vi "ziSweeperUtilEX.vi"(0 "Handle In":T1 {"Handle" format="0x%08x"; "Conn" format="0x%08x"}, 1 "Input Demods (0)":u16[](array[numeric])=[0], 2 "Oscillator (0)":u16, 3 "Order (4)":i32=4, 4 "Harmonic (1=fundamental)":i32=1 min=1 max=66000, 5 "Error In":errorcluster, 6 "Start (Hz)":dbl=10.0 format="%#_12p", 7 "average":u16, 8 "Stop (Hz)":dbl=10000.0 format="%#_12p", 9 "Precision (Low)":i32(ring)=5 items=["Low"=5, "Medium"=15, "High"=50], 10 "Steps (#)":i32=2, 11 "Min 1-w Damping (40dB)":dbl=40.0, 12 "Log Sweep (true)":bool=TRUE, 13 "Bandwith (-1=auto)":dbl=-1.0 format="%#_12p") -> (14 "Handle Out":T1 {"Handle" format="0x%08x"; "Conn" format="0x%08x"}, 15 "Output (F,X1,Y1,X2,Y2,...,Vo)":dbl[][](array[numeric]) format="%#_4p", 19 "Error Out":errorcluster)   [LabVIEW 2009, in "Zurich Instruments LabOne.lvlib"]
doc: "This utility configures an sweeper instance and returns after a complete single run the data recordered."
uses:
  <instrlib>/Zurich Instruments LabOne/Zurich Instruments LabOne.lvlib
  <instrlib>/Zurich Instruments LabOne/Public/ziTypeHandle.ctl
  <instrlib>/Zurich Instruments LabOne/Public/Modules/ziTypeModEnum.ctl
  <instrlib>/Zurich Instruments LabOne/Public/Modules/ziModSetValueDoubleArray.vi
  <instrlib>/Zurich Instruments LabOne/Public/Modules/ziModSetValueBinaryArray.vi
  <instrlib>/Zurich Instruments LabOne/Public/Configure/ziSetValueDouble.vi
  <instrlib>/Zurich Instruments LabOne/Public/Modules/ziModGetSweeperData.vi
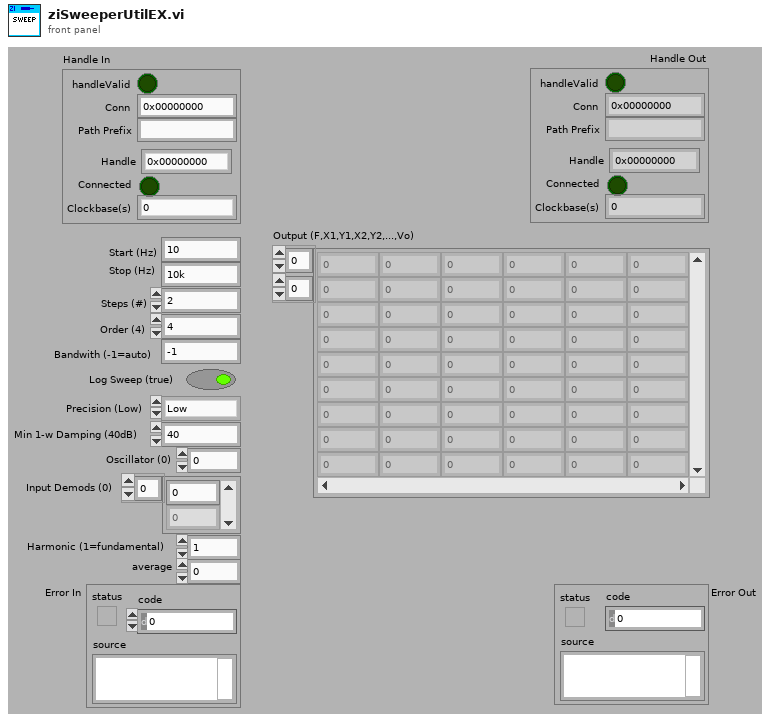
[diagram p1: front panel]
types:
  T1 = typedef "Zurich Instruments LabOne.lvlib/ziTypeHandle.ctl" = cluster{"handleValid":bool, "Conn":u64, "Path Prefix":string, "Handle":u64, "Connected":bool, "Clockbase(s)":dbl}
  T2 = typedef "Zurich Instruments LabOne.lvlib/ziTypeModEnum.ctl" = u16
  T3 = typedef "Zurich Instruments LabOne.lvlib/ziTypeModHandle.ctl" = cluster{"handleValid":bool, "Conn":u64, "ModHandle":u64, "moduleID":string, "Path Prefix":string}
  T4 = typedef "Zurich Instruments LabOne.lvlib/ziTypeModResults.ctl" = cluster{"PathArray":string[], "ValueType":T5, "NoOfResults":u64, "ziGenericHeader":T6[]}
  T5 = typedef "Zurich Instruments LabOne.lvlib/ziTypePollType.ctl" = enum16{"NONE", "DOUBLE_DATA", "INTEGER_DATA", "DEMOD_SAMPLE", "SCOPE_WAVE_HF2", "AUXIN_SAMPLE", "DIO_SAMPLE", "BYTE_ARRAY", "PWA_WAVE", "9", "10", "11", "12", "13", "14", "15", "TREE_CHANGE_DEPRI", "17", "ERROR", "19", "20", "21", "22", "23", "24", "25", "26", "27", "28", "29", "30", "31", "DOUBLE_DATA_TS", "INTEGER_DATA_TS", "34", "SCOPE_WAVE", "SCOPE_WAVE_EX", "37", "BYTE_ARRAY_TS", "39", "40", "41", "42", "43", "44", "45", "CNT_DATA", "47", "TREE_CHANGE", "49", "50", "51", "52", "53", "54", "55", "56", "57", "58", "59", "60", "61", "62", "63", "SWEEPER_DATA", "SPECTRUM_DATA", "ADVISOR_DATA", "VECTOR_DATA", "IMP_DATA"}
  T6 = typedef "Zurich Instruments LabOne.lvlib/ziTypeModGenericHeader.ctl" = cluster{"HeaderType":enum8{"HEADER_TYPE_NONE", "HEADER_TYPE_SWTRIGGER", "HEADER_TYPE_SWEEPER"}, "SampleFormat":u8, "SystemTime":timestamp, "CreatedTimeStamp":u64, "ChangedTimeStamp":u64, "Flags":u32, "ChunkSizeBytes":u64, "Name":string, "Status":u32, "GroupIndex":u32, "Color":u32, "ActiveRow":u32, "TriggerNumber":u64, "GridRows":u32, "GridCols":u32, "GridMode":u32, "GridOperation":u32, "GridDirection":u32, "GridRepetitions":u32, "GridColDelta":dbl, "GridColOffset":dbl, "GridRowDelta":dbl, "GridRowOffset":dbl, "Bandwidth":dbl, "Center":dbl, "Nenbw":dbl}
  T7 = typedef "Zurich Instruments LabOne.lvlib/ziTypeModSweeperDemodWave.ctl" = cluster{"timestamp":u64, "sampleCount":u64, "flags":u8, "sampleFormat":u8, "sweepMode":u8, "bandwidthMode":u8, "count":u64[], "settimestamp":u64[], "nexttimestamp":u64[], "grid":dbl[], "bandwidth":dbl[], "tc":dbl[], "tcmeas":dbl[], "settling":dbl[], "x":dbl[], "xstddev":dbl[], "xpwr":dbl[], "y":dbl[], "ystddev":dbl[], "ypwr":dbl[], "r":dbl[], "rstddev":dbl[], "rpwr":dbl[], "phase":dbl[], "phasestddev":dbl[], "phasepwr":dbl[], "frequency":dbl[], "frequencystddev":dbl[], "frequencypwr":dbl[], "auxin0":dbl[], "auxin0stddev":dbl[], "auxin0pwr":dbl[], "auxin1":dbl[], "auxin1stddev":dbl[], "auxin1pwr":dbl[]}
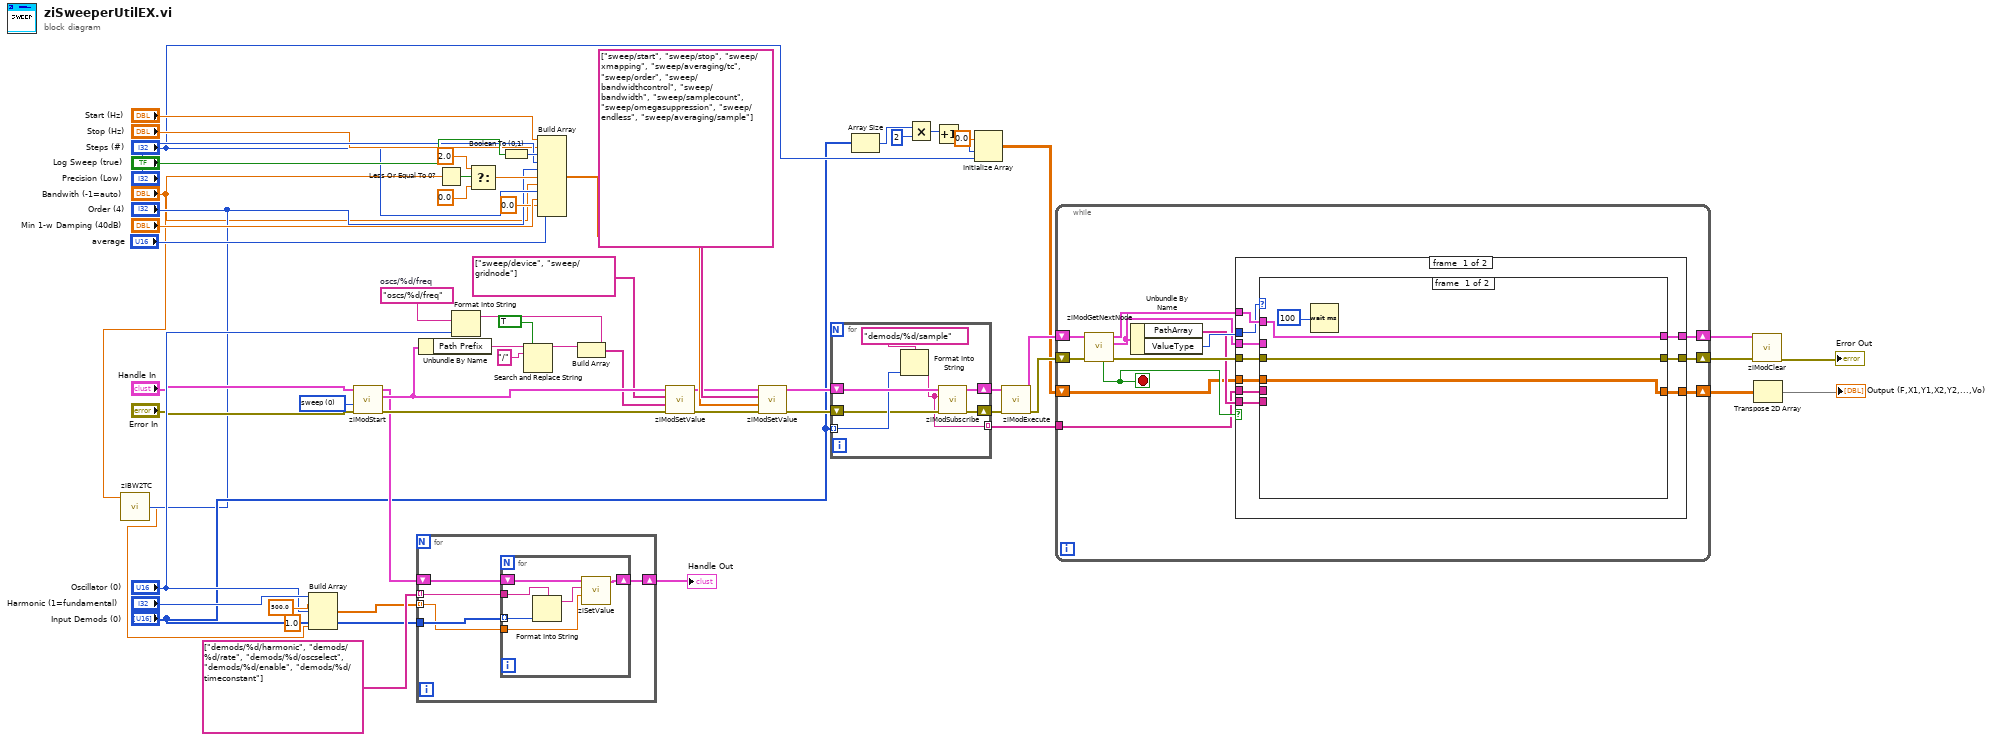
[diagram p0: block diagram]
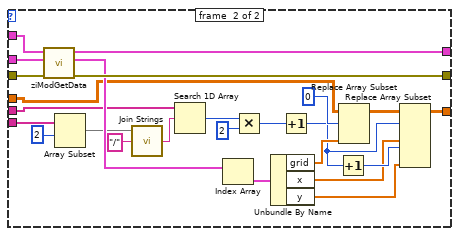
[diagram p2: hidden frame]
diagram:
  w1 = T2 0 items=["sweep", "scopeModule", "dataAcquisitionModule", "pidAdvisor", "awgModule", "impedanceModule", "multiDeviceSyncModule", "zoomFFT", "trigger", "deviceSettings", "record"] ("module Id")
  w23 = "oscs/%d/freq"  # oscs/%d/freq
  n1 = call <instrlib>:"ziBW2TC.vi"("Order (1)"="Order (4)", "BW (Hz)"="Bandwith (-1=auto)") -> ("TC (s)"=w2:dbl)  [unwired: 1 in]
  n2 = Build Array("Harmonic (1=fundamental)", 500.0 ("Value"), "Oscillator (0)", 1.0 ("element"), w2) -> (w36:dbl[])
  n3 = call <instrlib>:"ziModStart.vi"("Error In"="Error In", "module Id"=w1, "Handle In"="Handle In") -> ("Error Out"=w50:errorcluster, "ModHandle Out"=w43:T3, "Handle Out"=w35:T1)  [unwired: 6 in]
  n4 = for {
    tunnel: string[] ["demods/%d/harmonic", "demods/%d/rate", "demods/%d/oscselect", "demods/%d/enable", "demods/%d/timeconstant"] -> [w65] mode=indexing
    tunnel: "Input Demods (0)" -> [w64]
    tunnel: w36 -> [w63] mode=indexing
    shift-right: [w61] -> w26
    shift-left: w35 -> [w62]
    n5 = for {
      tunnel: w65 -> [w71]
      tunnel: w64 -> [w70] mode=indexing
      tunnel: w63 -> [w68]
      shift-right: [w66] -> w61
      shift-left: w62 -> [w67]
      n6 = Format Into String(format string=w71, w70) -> (resulting string=w69:string)  [unwired: 2 in, 1 out]
      n7 = call-poly <instrlib>:"ziSetValue.vi"("Value"=w68, "Path"=w69, "Handle In"=w67) -> ("Handle Out"=w66:T1)  [unwired: 2 in, 1 out]
    }
  }
  "Handle Out" <- w26
  n8 = Unbundle By Name(w43) -> ("Path Prefix"=w44:string)
  n9 = Less Or Equal To 0?(x="Bandwith (-1=auto)") -> (x <= 0?=w58:bool)
  n10 = Format Into String(format string=w23, "Oscillator (0)") -> (resulting string=w24:string)  [unwired: 2 in, 1 out]
  n11 = Select(t=2.0, s=w58, f=0.0) -> (s? t:f=w56:dbl)
  n12 = Boolean To (0,1)(Boolean="Log Sweep (true)") -> (0, 1=w59:i16)
  n13 = Search and Replace String(replace all?=TRUE ("replace all? (F)"), input string=w44, search string="/") -> (result string=w34:string)  [unwired: 5 in, 3 out]
  n14 = Build Array("Start (Hz)", "Stop (Hz)", w59, "Precision (Low)", "Order (4)", w56, "Bandwith (-1=auto)", "Steps (#)", "Min 1-w Damping (40dB)", 0.0 ("Value"), "average") -> (w54:dbl[])
  n15 = Build Array(w34, w24) -> (w32:string[])
  n16 = call-poly <instrlib>:"ziModSetValue.vi"("Error In"=w50, "Values"=w32, "Paths"=string[] ["sweep/device", "sweep/gridnode"], "ModHandle In"=w43) -> ("Error Out"=w30:errorcluster, "ModHandle Out"=w31:T3)  [unwired: 6 in]
  n17 = call-poly <instrlib>:"ziModSetValue.vi"("Error In"=w30, "Values"=w54, "Paths"=string[] ["sweep/start", "sweep/stop", "sweep/xmapping", "sweep/averaging/tc", "sweep/order", "sweep/bandwidthcontrol", "sweep/bandwidth", "sweep/samplecount", "sweep/omegasuppression", "sweep/endless", "sweep/averaging/sample"], "ModHandle In"=w31) -> ("Error Out"=w46:errorcluster, "ModHandle Out"=w47:T3)  [unwired: 6 in]
  n18 = for {
    tunnel: "Input Demods (0)" -> [w75] mode=indexing
    shift-right: [w78] -> w40
    shift-left: w46 -> [w74]
    shift-right: [w77] -> w41
    shift-left: w47 -> [w76]
    tunnel: [w72] -> w28 mode=indexing
    n19 = Format Into String(format string="demods/%d/sample", w75) -> (resulting string=w72:string)  [unwired: 2 in, 1 out]
    n20 = call <instrlib>:"ziModSubscribe.vi"("Error In"=w74, "Path"=w72, "ModHandle In"=w76) -> ("Error Out"=w78:errorcluster, "ModHandle Out"=w77:T3)  [unwired: 6 in]
  }
  n21 = Array Size(array="Input Demods (0)") -> (size(s)=w12:i32)
  n22 = Multiply(x=w12, y=2 ("index of element")) -> (x*y=w13:i32)
  n23 = Increment(x=w13) -> (x+1=w11:i32)
  n24 = Initialize Array(0.0 ("element"), w11, "Steps (#)") -> (w9:dbl[][])
  n25 = call <instrlib>:"ziModExecute.vi"("Error In"=w40, "ziModHandle In"=w41) -> ("Error Out"=w51:errorcluster, "ziModHandle Out"=w52:T3)  [unwired: 6 in, 1 out]
  n26 = while {
    shift-right: [w88] -> w48
    shift-left: w52 -> [w90]
    shift-right: [w87] -> w49
    shift-left: w51 -> [w91]
    tunnel: w28 -> [w81]
    shift-right: [w79] -> w18
    shift-left: w9 -> [w80]
    stop <- w85 stop-if-true
    n27 = call <instrlib>:"ziModGetNextNode.vi"("Error In"=w91, "ModHandle In"=w90) -> ("Error Out"=w86:errorcluster, "ModResults"=w83:T4, "ModHandle Out"=w89:T3, "NoData"=w85:bool)  [unwired: 6 in]
    n28 = Unbundle By Name(w83) -> ("PathArray"=w82:string[], "ValueType"=w84:T5)
    n29 = case shown="False" w85 {
      tunnel: w89 -> [w101 w132]
      tunnel: [w100 w132] -> w88
      tunnel: [w99 w133] -> w87
      tunnel: w86 -> [w98 w133]
      tunnel: w83 -> [w97 _]
      tunnel: w84 -> [w96 _]
      tunnel: w82 -> [w95 _]
      tunnel: w81 -> [w94 _]
      tunnel: w80 -> [w93 w131]
      tunnel: [w92 w131] -> w79
      frame #0 {
        n30 = case shown="\"NONE\", Default" w96 {
          tunnel: w101 -> [w105 w125]
          tunnel: w97 -> [_ w130]
          tunnel: w98 -> [w104 w129]
          tunnel: [w104 w128] -> w99
          tunnel: [w105 w127] -> w100
          tunnel: w95 -> [_ w120]
          tunnel: w94 -> [_ w119]
          tunnel: w93 -> [w102 w114]
          tunnel: [w102 w106] -> w92
          frame #0 {
            n31 = Wait (ms)(milliseconds to wait=u32 100) -> ()  [unwired: 1 out]
          }
          frame #1 {
            n32 = call-poly <instrlib>:"ziModGetData.vi"("Error In"=w129, "ModResults"=w130, "ModHandle In"=w125) -> ("Error Out"=w128:errorcluster, "SweeperDemodWaveArray"=w124:T7[], "ModHandle Out"=w127:T3)  [unwired: 4 in, 2 out]
            n33 = Array Subset(array=w120, index=2) -> (w122:string[])  [unwired: 1 in]
            n34 = call <vilib>:"Join Strings.vi"("Separator (,)"="/", "Strings In"=w122) -> ("String"=w118:string)  [unwired: 1 in]
            n35 = Search 1D Array(1D array=w119, element=w118) -> (index of element=w117:i32)  [unwired: 1 in]
            n36 = Index Array(array=w124) -> (element=w126:T7)  [unwired: 1 in]
            n37 = Multiply(x=w117, y=2 ("index of element")) -> (x*y=w115:i32)
            n38 = Unbundle By Name(w126) -> ("grid"=w112:dbl[], "x"=w108:dbl[], "y"=w107:dbl[])
            n39 = Increment(x=w115) -> (x+1=w110:i32)
            n40 = Increment(x=w110) -> (x+1=w109:i32)
            n41 = Replace Array Subset(array=w114, new element=w112, index (row)=0) -> (w111:dbl[][])  [unwired: 1 in]
            n42 = Replace Array Subset(array=w111, new element #1=w108, index (row) #1=w110, new element #2=w107, index (row) #2=w109) -> (w106:dbl[][])  [unwired: 2 in]
          }
        }
      }
      frame #1 {
      }
    }
  }
  n43 = call <instrlib>:"ziModClear.vi"("Error In"=w49, "ziModHandle In"=w48) -> ("Error Out"=→"Error Out":errorcluster)  [unwired: 7 in, 1 out]
  n44 = Transpose 2D Array(2D array=w18) -> (transposed array=→"Output (F,X1,Y1,X2,Y2,...,Vo)":dbl[][])
